vi "sendUpdatesDDS.vi"(7 "DDS: ProgramChanges":bool, 10 "Previous Ascii Array In":string[](array[string]), 11 "Current Ascii Array In":string[](array[string])) -> (2 "Last written Ascii array Out":string[](array[string]), 3 "Current Ascii Array Out":string[](array[string]))   [LabVIEW 2013, in "DDS9954_v2013.lvlib"]
uses:
  DDS9954_v2013.lvlib
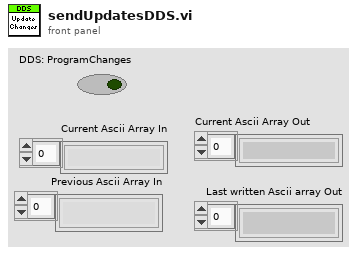
[diagram p1: front panel]
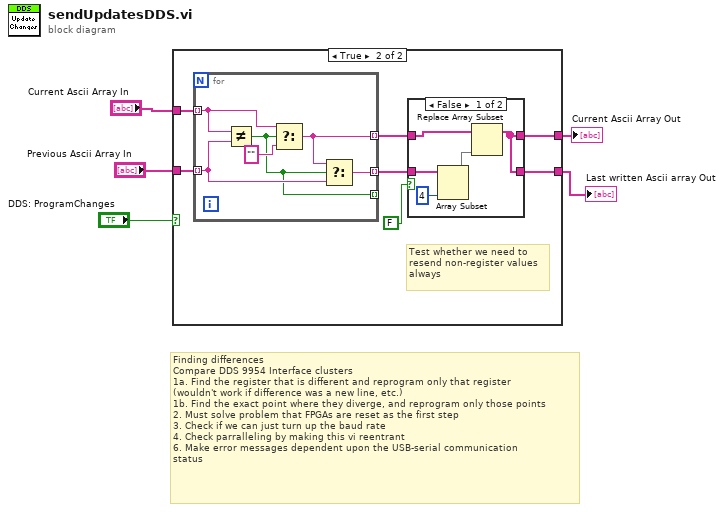
[diagram p0: block diagram]
diagram:
  # "Finding differences\nCompare DDS 9954 Interface clusters\n1a. Find the register that is different and reprogram only that register\n(wouldn't work if difference was a new line, etc.)\n1b. Find the exact point where they diverge, and reprogram only those points\n2. Must solve problem that FPGAs are reset as the first step\n3. Check if we can just turn up the baud rate\n4. Check parralleling by making this vi reentrant\n6. Make error messages dependent upon the USB-serial communication\nstatus"
  n1 = case shown="True" "DDS: ProgramChanges" {
    tunnel: "Current Ascii Array In" -> [w6 w13]
    tunnel: "Previous Ascii Array In" -> [_ w12]
    tunnel: [w6 w7] -> w4
    tunnel: [w6 w8] -> w2
    frame False {
    }
    frame True {
      # "Test whether we need to\nresend non-register values\nalways"
      n2 = for {
        tunnel: w13 -> [w26] mode=indexing
        tunnel: w12 -> [w23] mode=indexing
        tunnel: [w24] -> w11 mode=indexing
        tunnel: [w22] -> w10 mode=indexing
        tunnel: [w21] -> _ mode=indexing
        n3 = Not Equal?(x=w26, y=w23) -> (x != y?=w21:bool)
        n4 = Select(t=w26, s=w21, f="") -> (s? t:f=w24:string)
        n5 = Select(t=w24, s=w21, f=w23) -> (s? t:f=w22:string)
      }
      n6 = case shown="False" FALSE {
        tunnel: w11 -> [w15 w20]
        tunnel: w10 -> [w18 w19]
        tunnel: [w14 w20] -> w8
        tunnel: [w14 w19] -> w7
        frame False {
          n7 = Array Subset(array=w18, length=4) -> (w16:string[])  [unwired: 1 in]
          n8 = Replace Array Subset(array=w15, new element=w16) -> (w14:string[])  [unwired: 1 in]
        }
        frame True {
        }
      }
    }
  }
  "Last written Ascii array Out" <- w4
  "Current Ascii Array Out" <- w2
